vi "Modify_Metadata_Channels.vi"(4 "Ch Description Array":T1[](array[typedef]) {"Duty" format="%.0b"; "D" format="%#_5g"; "C" format="%#_5g"; "B" format="%#_5g"; "A" format="%#_5g"}) -> (1 "Ch Description Array Out":T1[](array[typedef]) {"Duty" format="%.0b"; "D" format="%#_5g"; "C" format="%#_5g"; "B" format="%#_5g"; "A" format="%#_5g"})   [LabVIEW 2013]
uses:
  ADAM Controls/Ch_description_ADAM.ctl
  ADAM Controls/Module_type_ADAM.ctl
  ADAM Controls/Function_ADAM.ctl
  ADAM Controls/Channel_State.ctl
  ADAM Controls/Calib_type_ADAM.ctl
  ADAM Controls/Address.ctl
  Anemometry/Anemometry Sub Vis/Globals/Preference_global.vi
panel:
  in  "Cluster Template":cluster{"Channel Name":string, "Menu Ring":bool}
  in  "Channel Types":T7(array[cluster])
  in  "Select Channels to Activate":i32[](listbox)
  in  "Add a New Channel":bool
  in  "stop":bool
  in  "OK":bool
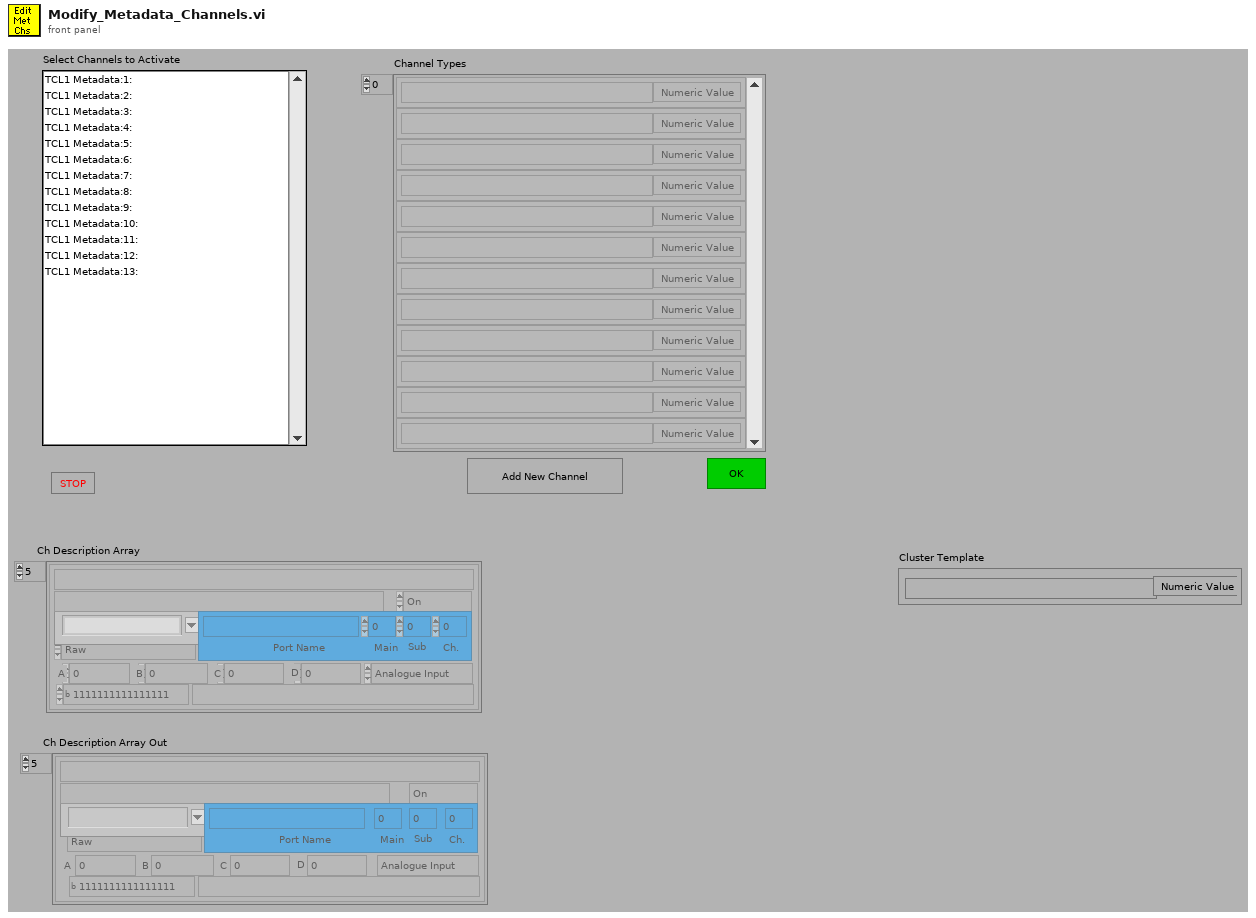
[diagram p1: front panel]
types:
  T1 = typedef "Ch_description_ADAM.ctl" = cluster{"Ch Name":string, "Type":T2, "Function":T3, "Ch State":T4, "Calibration type":T5, "A":dbl, "B":dbl, "C":dbl, "D":dbl, "Comments":string, "Address":T6, "String":string, "Duty":u16}
  T2 = typedef "Module_type_ADAM.ctl" = string
  T3 = typedef "Function_ADAM.ctl" = enum16{"Analogue Input", "Digital Input", "Event counter", "Event rate", "Analogue Output", "Digital Output", "Relay Output"}
  T4 = typedef "Channel_State.ctl" = enum16{"On", "Off", "Always On", "Always Off"}
  T5 = typedef "Calib_type_ADAM.ctl" = enum16{"Raw", "Bx + A", "Cx^2 + Bx + A", "Dx^3 + Cx^2 + Bx + A", "In Band", "Hi-Tec Q", "Hi-Tec M_dot", "Text"}
  T6 = typedef "Address.ctl" = cluster{"Main":i32, "Ch.":i32, "Sub":i32, "Port Name":string}
  T7 = cluster{"Channel Name":string, "Menu Ring":bool}[]
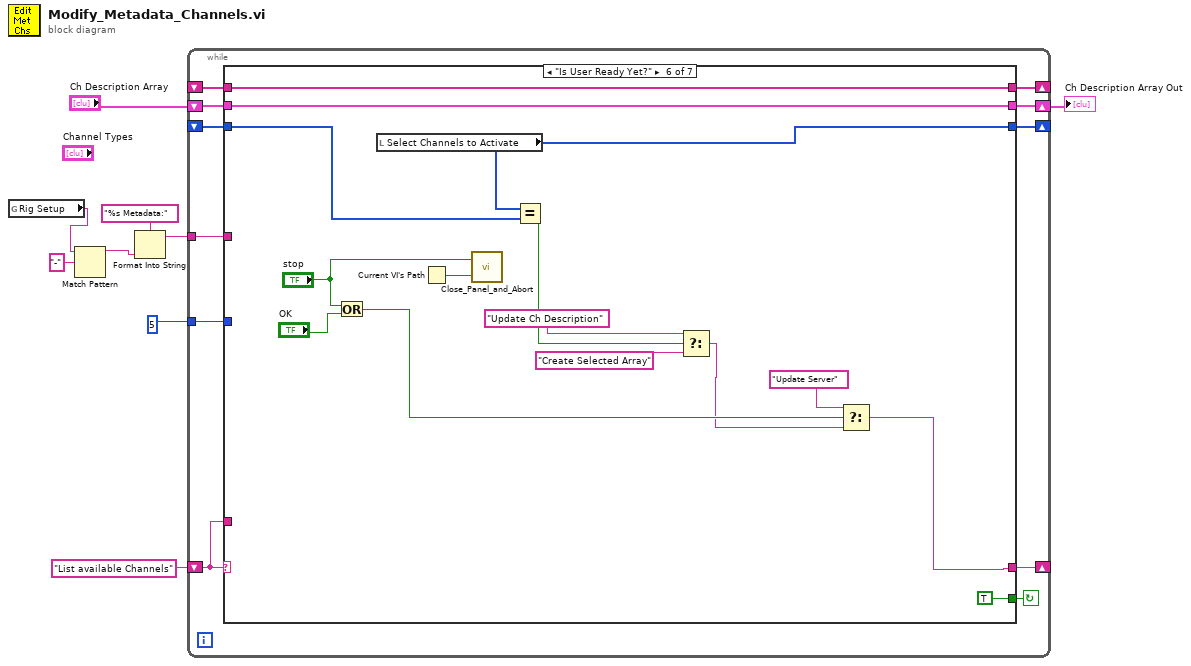
[diagram p0: block diagram]
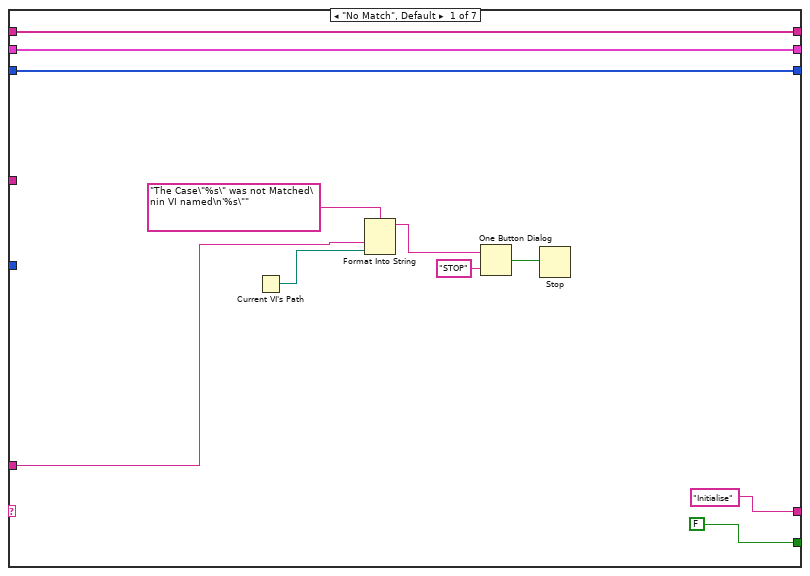
[diagram p2: hidden frame]
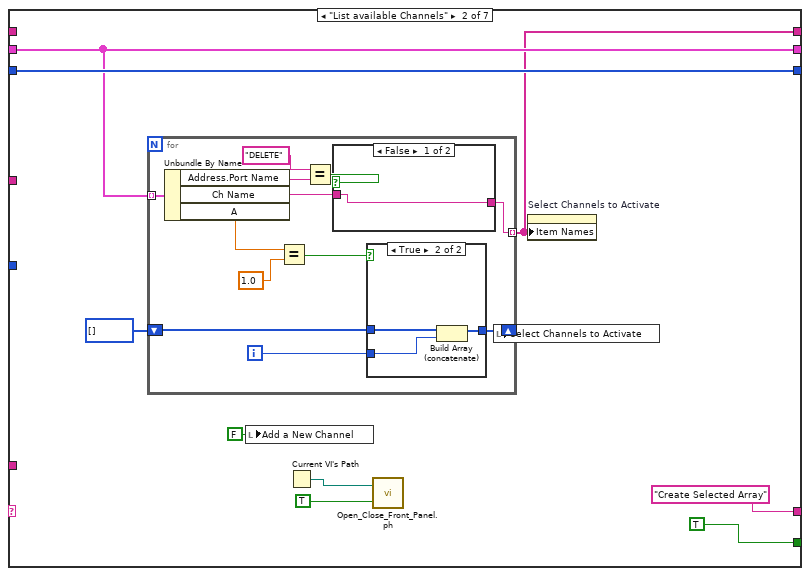
[diagram p3: hidden frame]
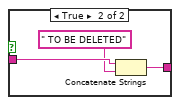
[diagram p4: hidden frame]
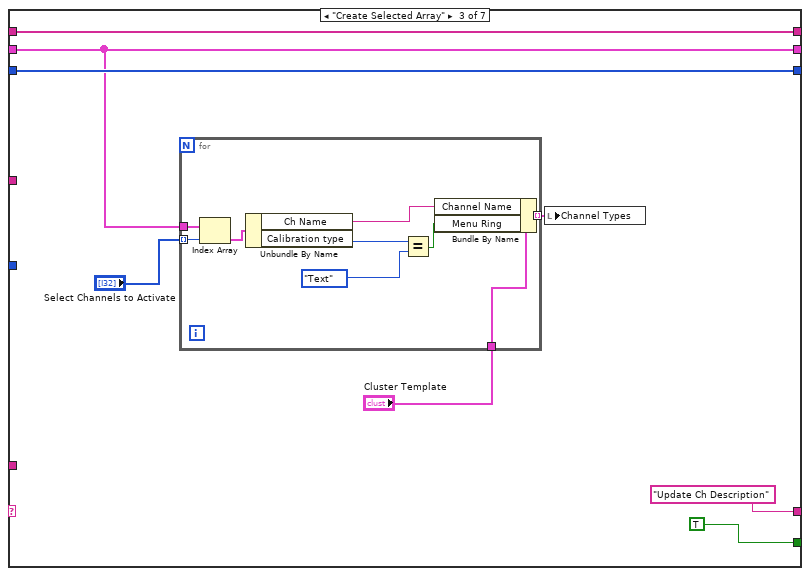
[diagram p6: hidden frame]
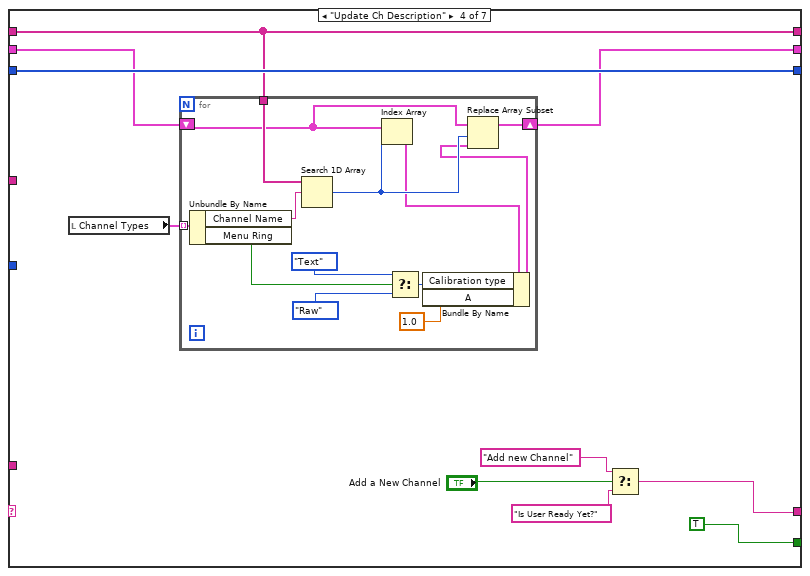
[diagram p7: hidden frame]
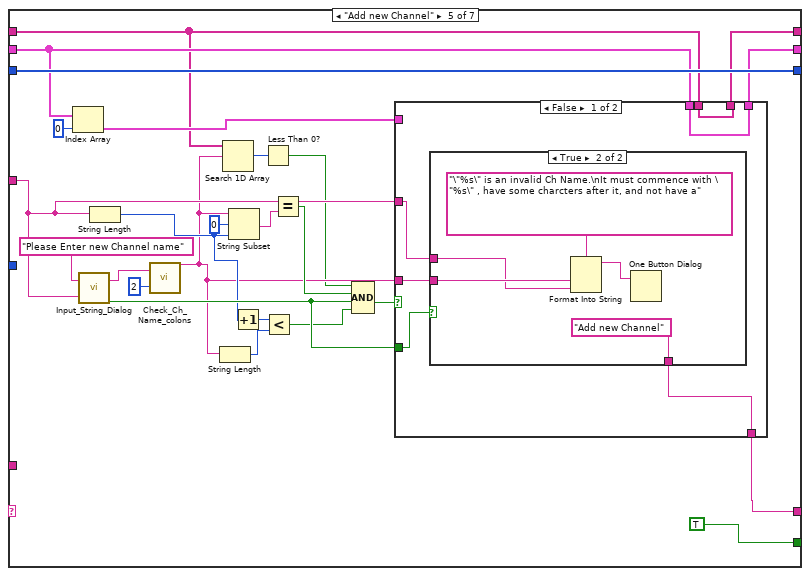
[diagram p8: hidden frame]
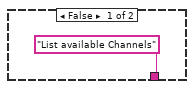
[diagram p9: hidden frame]
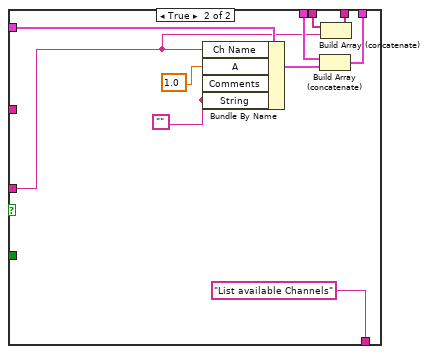
[diagram p10: hidden frame]
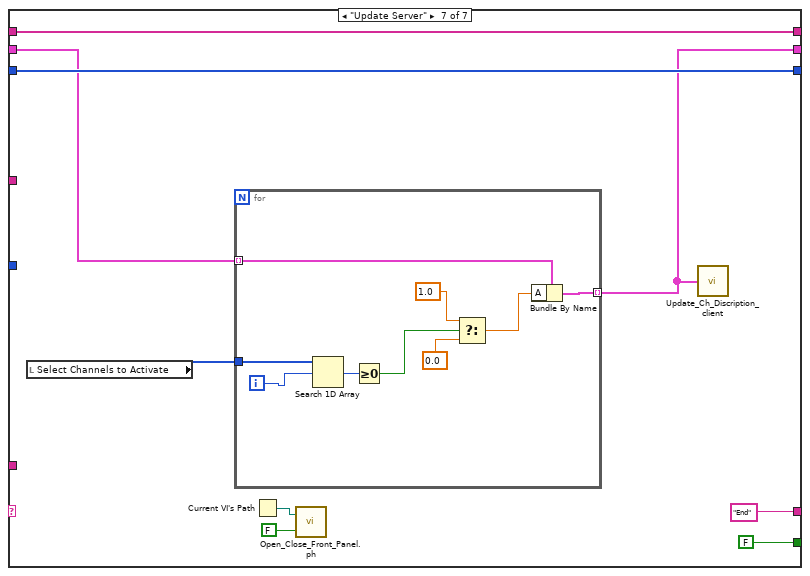
[diagram p11: hidden frame]
diagram:
  n1 = global read "Preference_global.vi" "Rig Setup"() -> (w2:string)
  n2 = Match Pattern(string=w2, regular expression="-") -> (before substring=w1:string)  [unwired: 4 out]
  n3 = Format Into String(format string="%s Metadata:" ("Format String"), w1) -> (resulting string=w7:string)  [unwired: 2 in, 1 out]
  n4 = while {
    tunnel: 5 -> [w10]
    tunnel: w7 -> [w11]
    shift-left: _ -> [w14]
    shift-right: [w13] -> _
    shift-left: _ -> [w15]
    shift-right: [w17] -> _
    shift-left: "Ch Description Array" -> [w16]
    shift-right: [w18] -> w4
    shift-left: "List available Channels" -> [w19]
    shift-right: [w12] -> _
    stop <- w20 continue-if-true
    n5 = case shown="\"Is User Ready Yet?\"" w19 {
      tunnel: [FALSE TRUE TRUE TRUE TRUE TRUE ("T button?") FALSE ("T button?")] -> w20
      tunnel: ["Initialise" "Create Selected Array" "Update Ch Description" w79 w113 w149 "End"] -> w12
      tunnel: w19 -> [w26 _ _ _ _ _ _]
      tunnel: [w23 w38 w65 w85 w121 w163 w166] -> w18
      tunnel: [w22 w39 w67 w87 w125 w157 w169] -> w17
      tunnel: w16 -> [w23 w38 w65 w84 w120 w163 w168]
      tunnel: w15 -> [w22 w39 w67 w87 w125 w156 w169]
      tunnel: w14 -> [w21 _ w62 w83 w105 w158 w170]
      tunnel: [w21 w35 w62 w83 w119 w158 w170] -> w13
      tunnel: w11 -> [_ _ _ _ w114 _ _]
      tunnel: w10 -> [_ _ _ _ _ _ _]
      frame "No Match", Default {
        n6 = Current VI's Path() -> (path=w25:path)
        n7 = Format Into String(format string="The Case\"%s\" was not Matched\nin VI named\n'%s\"" ("Format String"), w26, w25) -> (resulting string=w29:string)  [unwired: 2 in, 1 out]
        n8 = One Button Dialog(message=w29, button name ("OK")="STOP") -> (true=w27:bool)
        n9 = Stop(stop? (T)=w27) -> ()
      }
      frame "List available Channels" {
        n10 = for {
          tunnel: w38 -> [w53] mode=indexing
          tunnel: [w42] -> w35 mode=indexing
          shift-right: [w48] -> w36
          shift-left: i32[] [] -> [w49]
          i -> [w47]
          n11 = Unbundle By Name(w53) -> ("Address.Port Name"=w46:string, "Ch Name"=w43:string, "A"=w52:dbl)
          n12 = Equal?(x=w52, y=1.0) -> (x = y?=w50:bool)
          n13 = Equal?(x="DELETE", y=w46) -> (x = y?=w44:bool)
          n14 = case shown="False" w44 {
            tunnel: w43 -> [w54 w57]
            tunnel: [w54 w55] -> w42
            frame False {
            }
            frame True {
              n15 = Concatenate Strings(w57, " TO BE DELETED" ("string")) -> (w55:string)
            }
          }
          n16 = case shown="True" w50 {
            tunnel: w49 -> [w58 w61]
            tunnel: [w58 w60] -> w48
            tunnel: w47 -> [_ w59]
            frame False {
            }
            frame True {
              n17 = Build Array (concatenate)(w61, w59) -> (w60:i32[])
            }
          }
        }
        n18 = local write "Add a New Channel"(FALSE ("Add a New Channel")) -> ()
        n19 = Current VI's Path() -> (path=w33:path)
        n20 = call "Open_Close_Front_Panel.ph.vi"("Front Panel Window:Open"=TRUE, "VI path"=w33) -> ()  [unwired: 2 out]
        n21 = local write "Select Channels to Activate"(w36) -> ()
        n22 = property on="Select Channels to Activate" class="LstBox (strict)"("Item Names"=w35) -> ()  [unwired: 2 in, 2 out]
      }
      frame "Create Selected Array" {
        n23 = for {
          tunnel: "Select Channels to Activate" -> [w78] mode=indexing
          tunnel: w65 -> [w77]
          tunnel: "Cluster Template" -> [w73]
          tunnel: [w70] -> w63 mode=indexing
          n24 = Index Array(array=w77, index=w78) -> (element=w76:T1)
          n25 = Unbundle By Name(w76) -> ("Ch Name"=w71:string, "Calibration type"=w75:T5)
          n26 = Equal?(x=w75, y=Calib_type_ADAM."Text" ("Calibration Type")) -> (x = y?=w72:bool)
          n27 = Bundle By Name(cluster=w73, "Channel Name"=w71, "Menu Ring"=w72) -> (w70:cluster{"Channel Name":string, "Menu Ring":bool})
        }
        n28 = local write "Channel Types"(w63) -> ()
      }
      frame "Update Ch Description" {
        n29 = local read "Channel Types"() -> (w86:T7)
        n30 = for {
          tunnel: w86 -> [w101] mode=indexing
          tunnel: w83 -> [w100]
          shift-right: [w93] -> w85
          shift-left: w84 -> [w94]
          n31 = Unbundle By Name(w101) -> ("Channel Name"=w99:string, "Menu Ring"=w98:bool)
          n32 = Search 1D Array(1D array=w100, element=w99) -> (index of element=w95:i32)  [unwired: 1 out]
          n33 = Index Array(array=w94, index=w95) -> (element=w92:T1)
          n34 = Select(t=Calib_type_ADAM."Text" ("Calibration Type"), s=w98, f=Calib_type_ADAM."Raw" ("Calibration Type")) -> (s? t:f=w91:T5)
          n35 = Bundle By Name(cluster=w92, "Calibration type"=w91, "A"=1.0 ("Bundle Element")) -> (w89:T1)
          n36 = Replace Array Subset(array=w94, new element=w89, index=w95) -> (w93:T1[])
        }
        n37 = Select(t="Add new Channel", s="Add a New Channel", f="Is User Ready Yet?") -> (s? t:f=w79:string)
      }
      frame "Add new Channel" {
        n38 = Index Array(array=w120, index=0 ("Index")) -> (element=w123:T1)
        n39 = call "Input_String_Dialog.vi"("Value"=w114, "Message to user"="Please Enter new Channel name") -> ("Ok Out"=w112:bool, "Output string"=w111:string)
        n40 = String Length(string=w114) -> (length=w108:i32)
        n41 = call "Check_Ch_Name_colons.vi"("No of Colons"=2, "Ch Name in"=w111) -> ("Ch Name out"=w104:string)
        n42 = String Length(string=w104) -> (length=w109:i32)
        n43 = Search 1D Array(1D array=w105, element=w104) -> (index of element=w103:i32)  [unwired: 1 out]
        n44 = String Subset(string=w104, offset (0)=0, length (rest)=w108) -> (substring=w117:string)
        n45 = Increment(x=w108) -> (x+1=w107:i32)
        n46 = Less Than 0?(x=w103) -> (x < 0?=w102:bool)
        n47 = Less?(x=w107, y=w109) -> (x < y?=w106:bool)
        n48 = Equal?(x=w114, y=w117) -> (x = y?=w116:bool)
        n49 = Compound Arithmetic op=AND(w102, w116, w112, w106) -> (w115:bool)
        n50 = case shown="False" w115 {
          tunnel: w104 -> [w130 w142]
          tunnel: w123 -> [_ w148]
          tunnel: w120 -> [w132 w146]
          tunnel: [w132 w145] -> w121
          tunnel: w105 -> [w131 w144]
          tunnel: [w131 w143] -> w119
          tunnel: w114 -> [w129 _]
          tunnel: [w127 "List available Channels"] -> w113
          tunnel: w112 -> [w128 _]
          frame False {
            n51 = case shown="True" w128 {
              tunnel: w130 -> [_ w138]
              tunnel: w129 -> [_ w136]
              tunnel: ["List available Channels" "Add new Channel"] -> w127
              frame False {
              }
              frame True {
                n52 = Format Into String(format string="\"%s\" is an invalid Ch Name.\nIt must commence with \"%s\" , have some charcters after it, and not have a" ("Format String"), w138, w136) -> (resulting string=w135:string)  [unwired: 2 in, 1 out]
                n53 = One Button Dialog(message=w135) -> ()  [unwired: 2 out]
              }
            }
          }
          frame True {
            w139 = ""
            n54 = Bundle By Name(cluster=w148, "Ch Name"=w142, "A"=1.0 ("Bundle Element"), "Comments"=w139, "String"=w139) -> (w147:T1)
            n55 = Build Array (concatenate)(w146, w147) -> (w145:T1[])
            n56 = Build Array (concatenate)(w144, w142) -> (w143:string[])
          }
        }
      }
      frame "Is User Ready Yet?" {
        n57 = Or(x="stop", y="OK") -> (x .or. y?=w152:bool)
        n58 = local read "Select Channels to Activate"() -> (w157:i32[])
        n59 = Current VI's Path() -> (path=w162:path)
        n60 = call "Close_Panel_and_Abort.vi"("Vi path"=w162, "stop"="stop") -> ()  [unwired: 1 out]
        n61 = Equal?(x=w157, y=w156) -> (x = y?=w154:bool)
        n62 = Select(t="Update Ch Description", s=w154, f="Create Selected Array") -> (s? t:f=w151:string)
        n63 = Select(t="Update Server", s=w152, f=w151) -> (s? t:f=w149:string)
      }
      frame "Update Server" {
        n64 = local read "Select Channels to Activate"() -> (w167:i32[])
        n65 = for {
          tunnel: w168 -> [w179] mode=indexing
          tunnel: w167 -> [w181]
          tunnel: [w178] -> w166 mode=indexing
          i -> [w180]
          n66 = Search 1D Array(1D array=w181, element=w180) -> (index of element=w177:i32)  [unwired: 1 out]
          n67 = Greater Or Equal To 0?(x=w177) -> (x >= 0?=w176:bool)
          n68 = Select(t=1.0, s=w176, f=0.0 ("Bundle Element")) -> (s? t:f=w173:dbl)
          n69 = Bundle By Name(cluster=w179, "A"=w173) -> (w178:T1)
        }
        n70 = Current VI's Path() -> (path=w165:path)
        n71 = call "Open_Close_Front_Panel.ph.vi"("Front Panel Window:Open"=FALSE, "VI path"=w165) -> ()  [unwired: 2 out]
        n72 = call "Update_Ch_Discription_client.vi"("Channels to update In"=w166) -> ()  [unwired: 1 out]
      }
    }
  }
  "Ch Description Array Out" <- w4
